vi "Right LIDAR Loop (SubVI).vi"(11 "Refnum in":refnum<k20>) -> ()   [LabVIEW 2015]
uses:
  Right Variables.vi
  <vilib>/Utility/error.llb/Error Cluster From Error Code.vi
  <vilib>/rvi/errors/niLvFpgaAdjustHostInterfaceError.vi
  <vilib>/FPGAPlugInAG/Dynamic/niLvFpga_Close_Dynamic.vi
  <vilib>/rvi/interface/nirviReadWriteControl/nirviReadWriteControl.xnode
  <vilib>/rvi/interface/nirviCloseFPGA/nirviCloseFPGA.xnode
  NiFpgaLv.dll
  <vilib>/rvi/interface/Simulation/niFpgaSimulationCallBeginRW.vi
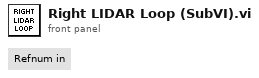
[diagram p1: front panel]
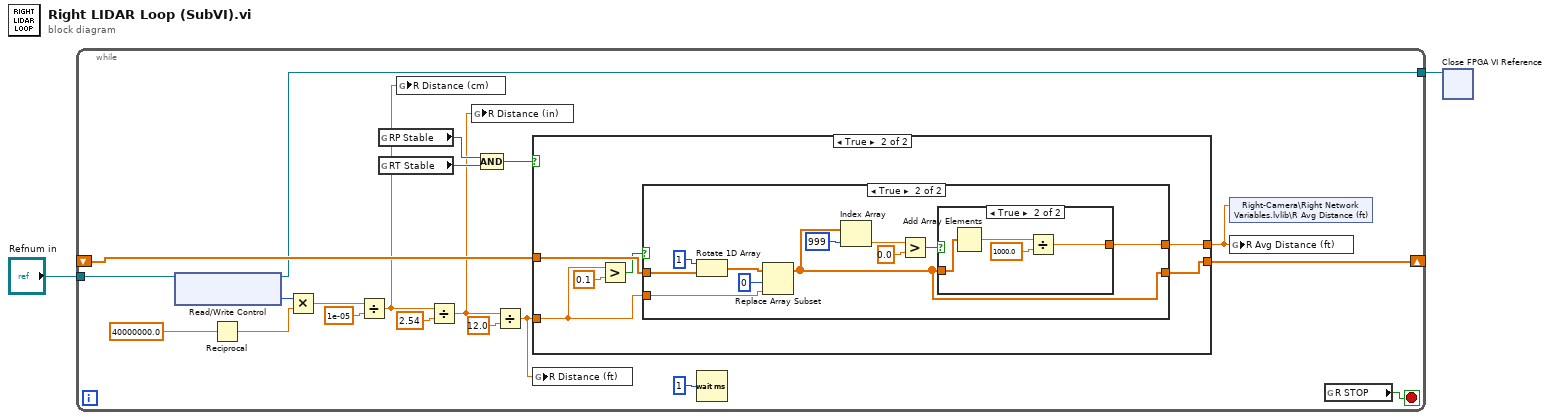
[diagram p0: block diagram]
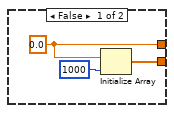
[diagram p2: hidden frame]
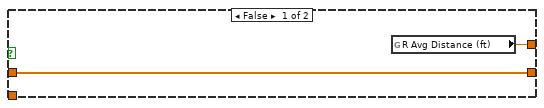
[diagram p3: hidden frame]
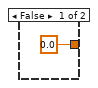
[diagram p4: hidden frame]
diagram:
  n1 = while {
    tunnel: "Refnum in" -> [w7]
    tunnel: [w8] -> w2
    shift-right: [w21] -> _
    shift-left: _ -> [w20]
    stop <- w18 stop-if-true
    n2 = xnode "Read/Write Control"("FPGA VI Reference In"=w7) -> ("FPGA VI Reference Out"=w8:refnum<k20>, "Pulse width ticks"=w11:u32)  [unwired: 1 in, 1 out]
    n3 = Reciprocal(x=40000000.0) -> (1/x=w10:dbl)
    n4 = Multiply(x=w11, y=w10) -> (x*y=w12:dbl)
    n5 = Divide(x=w12, y=1e-05) -> (x/y=w6:dbl)
    n6 = global read "Right Variables.vi" "RP Stable"() -> (w17:bool)
    n7 = global read "Right Variables.vi" "RT Stable"() -> (w16:bool)
    n8 = global write "Right Variables.vi" "R Distance (cm)"(w6) -> ()
    n9 = Divide(x=w6, y=2.54) -> (x/y=w5:dbl)
    n10 = global write "Right Variables.vi" "R Distance (in)"(w5) -> ()
    n11 = Compound Arithmetic op=AND(w17, w16) -> (w22:bool)
    n12 = Divide(x=w5, y=12.0) -> (x/y=w4:dbl)
    n13 = case shown="True" w22 {
      tunnel: w20 -> [_ w31]
      tunnel: [w23 w29] -> w21
      tunnel: [w24 w30] -> w3
      tunnel: w4 -> [_ w27]
      frame False {
        w24 = 0.0 ("element")
        n14 = Initialize Array(w24, 1000 ("dimension size")) -> (w23:dbl[])
      }
      frame True {
        n15 = Greater?(x=w27, y=0.1) -> (0:w26:bool)
        n16 = case shown="True" w26 {
          tunnel: w31 -> [w32 w37]
          tunnel: [w33 w36] -> w30
          tunnel: [w32 w35] -> w29
          tunnel: w27 -> [_ w34]
          frame False {
            n17 = global read "Right Variables.vi" "R Avg Distance (ft)"() -> (w33:dbl)
          }
          frame True {
            n18 = Rotate 1D Array(1:w37, 2:1 ("n")) -> (0:w43:dbl[])
            n19 = Replace Array Subset(array=w43, new element=w34, index=0) -> (w35:dbl[])
            n20 = Index Array(array=w35, index=999) -> (element=w40:dbl)
            n21 = Greater?(x=w40, y=0.0) -> (0:w38:bool)
            n22 = case shown="True" w38 {
              tunnel: w35 -> [_ w49]
              tunnel: [0.0 w46] -> w36
              frame False {
              }
              frame True {
                n23 = Add Array Elements(numeric array=w49) -> (sum=w48:dbl)
                n24 = Divide(x=w48, y=1000.0) -> (x/y=w46:dbl)
              }
            }
          }
        }
      }
    }
    n25 = global write "Right Variables.vi" "R Distance (ft)"(w4) -> ()
    n26 = Wait (ms)(milliseconds to wait=u32 1) -> ()  [unwired: 1 out]
    n27 = shared-variable "Right-Camera\\Right Network Variables.lvlib\\R Avg Distance (ft)"(w3) -> ()  [unwired: 1 in, 1 out]
    n28 = global write "Right Variables.vi" "R Avg Distance (ft)"(w3) -> ()
    n29 = global read "Right Variables.vi" "R STOP"() -> (w18:bool)
  }
  n30 = xnode "Close FPGA VI Reference"("FPGA VI Reference In"=w2) -> ()  [unwired: 1 in, 1 out]
